vi "GET_security_acces_seed_and_key.vi"(8 "API Key":string="cheia04042025tema2restfulapi") -> (0 "key":u64, 1 "seed":u64, 2 "headers":string, 3 "error out json":errorcluster, 4 "body":string, 5 "error out get":errorcluster)   [LabVIEW 2024]
uses:
  <vilib>/httpClient/LabVIEWHTTPClient.lvlib
panel:
  # "INPUTS"
  # "OUTPUTS"
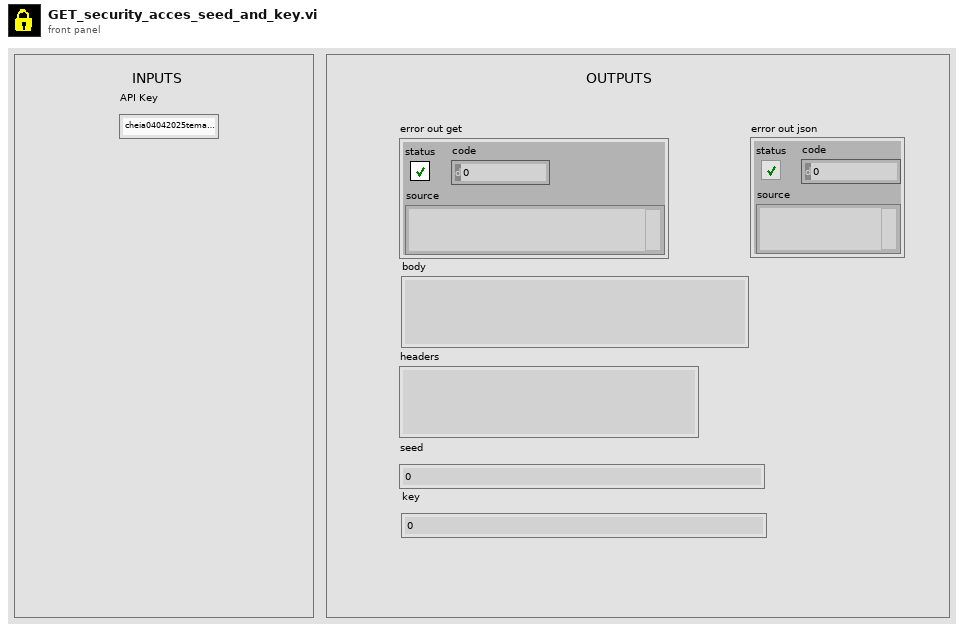
[diagram p1: front panel]
types:
  T1 = typedef "LabVIEWHTTPClient.lvlib/ClientHandle.ctl" = refnum<k1>
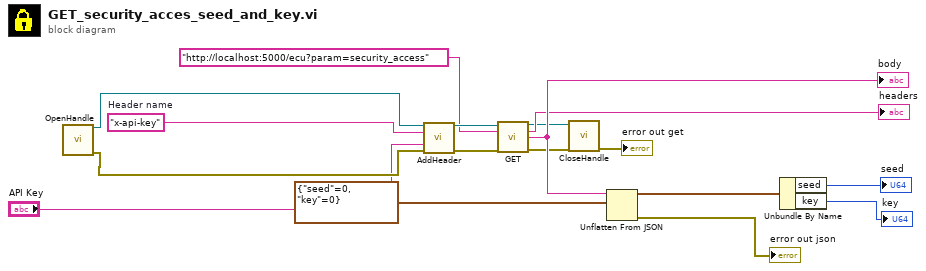
[diagram p0: block diagram]
diagram:
  w3 = "x-api-key"  # Header name
  n1 = call <vilib>:"OpenHandle.vi"() -> ("client handle out"=w5:T1, "error out"=w6:errorcluster)  [unwired: 14 in]
  n2 = call <vilib>:"AddHeader.vi"("client handle"=w5, "header"=w3, "value"="API Key", "error in (no error)"=w6) -> ("client handle out"=w8:T1, "error out"=w7:errorcluster)  [unwired: 10 in]
  n3 = call <vilib>:"GET.vi"("client handle"=w8, "url"="http://localhost:5000/ecu?param=security_access", "error in (no error)"=w7) -> ("client handle out"=w10:T1, "headers"=→"headers":string, "body"=w17:string, "error out"=w9:errorcluster)  [unwired: 9 in]
  "body" <- w17
  n4 = call <vilib>:"CloseHandle.vi"("client handle"=w10, "error in (no error)"=w9) -> ("error out"=→"error out get":errorcluster)  [unwired: 13 in]
  n5 = Unflatten From JSON(JSON string=w17, type and defaults=cluster{"seed":u64, "key":u64} {"seed"=0, "key"=0}) -> (value=w14:cluster{"seed":u64, "key":u64}, error out=→"error out json":errorcluster)  [unwired: 5 in]
  n6 = Unbundle By Name(w14) -> ("seed"=→"seed":u64, "key"=→"key":u64)
